vi "Generate write queue item.vi"(8 "error in (no error)":errorcluster, 9 "Subscription ID":u64, 10 "Request ID":u64, 11 "Unsubscribe JSON in":refnum<class "Unsubscribe JSON.lvclass">) -> (0 "error out":errorcluster, 2 "Write queue item":T1, 3 "Unsubscribe JSON out":refnum<class "Unsubscribe JSON.lvclass">)   [LabVIEW 2020, in "wamplv.lvlib" / "Unsubscribe JSON.lvclass"]
uses:
  Unsubscribe JSON.lvclass
  Unsubscribe JSON.lvclass/Unsubscribe JSON.ctl
  wamplv.lvlib
  TypeDefs/WAMP Message Codes.ctl
  fa963b5a-339b-4bff-adac-c53375f7ee2f.vi
  TypeDefs/Transport type.ctl
  WAMP Client/Private/TypeDef/Write queue item.ctl
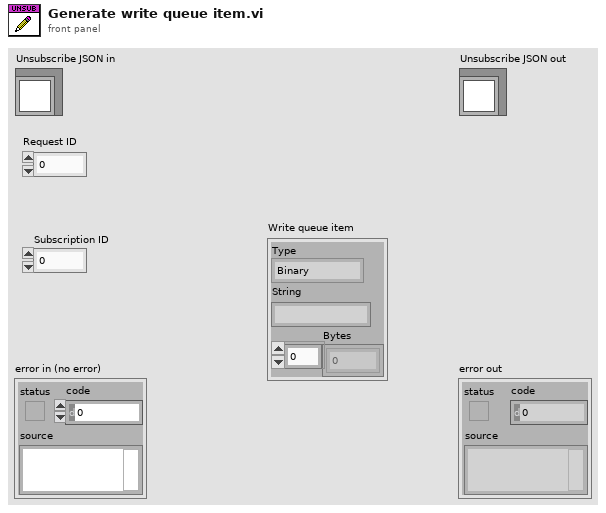
[diagram p1: front panel]
types:
  T1 = typedef "wamplv.lvlib/Write queue item.ctl" = cluster{"Type":T2, "String":string, "Bytes":u8[]}
  T2 = typedef "wamplv.lvlib/Transport type.ctl" = enum16{"Binary", "Text"}
  T3 = typedef "wamplv.lvlib/WAMP Message Codes.ctl" = enum8{"HELLO", "WELCOME", "ABORT", "GOODBYE", "ERROR", "PUBLISH", "PUBLISHED", "SUBSCRIBE", "SUBSCRIBED", "UNSUBSCRIBE", "UNSUBSCRIBED", "EVENT", "CALL", "RESULT", "REGISTER", "REGISTERED", "UNREGISTER", "UNREGISTERED", "INVOCATION", "YIELD"}
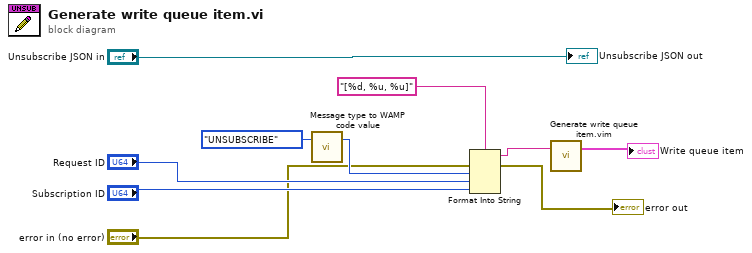
[diagram p0: block diagram]
diagram:
  n1 = call "Message type to WAMP code value.vi"("Message Type"=WAMP_Message_Codes."UNSUBSCRIBE") -> ("WAMP Numeric value"=w5:u8)  [unwired: 2 in]
  n2 = Format Into String(format string="[%d, %u, %u]" ("element"), error in="error in (no error)", w5, "Request ID", "Subscription ID") -> (resulting string=w2:string, error out=→"error out":errorcluster)  [unwired: 1 in]
  n3 = call "Generate write queue item.vim"("Input"=w2) -> ("Ouput"=→"Write queue item":T1)  [unwired: 2 in]
  "Unsubscribe JSON out" <- "Unsubscribe JSON in"
